vi "Node Status to gRPC Status.vi"(2 "Node Status":T10 {"Monitor Doubles"."4" format="%#_9g"; "Monitor Doubles"."3" format="%#_9g"; "Monitor Doubles"."2" format="%#_9g"; "Monitor Doubles"."1" format="%#_9g"}) -> (4 "gRPC Status":T1)   [LabVIEW 2021, in "CIFCoreCommon.lvlib"]
uses:
  CIFCoreCommon.lvlib
  Typedef/Plugin Status.ctl
  Typedef/Plugin State.ctl
  Typedef/Timing Statistics.ctl
  Typedef/Timing Stats Base.ctl
  Typedef/FIFO Statistics.ctl
  Typedef/Simple Error.ctl
  Typedef/Monitor Doubles.ctl
  Typedef/Monitor U64.ctl
  Typedef/Monitor I64.ctl
  Grpc/CIFCorePlugin_client/RPC Messages/cif_plugincore_StatusData.ctl
  Grpc/CIFCorePlugin_client/RPC Messages/cif_plugincore_StatusData_State.ctl
  Grpc/CIFCorePlugin_client/RPC Messages/cif_plugincore_TimingStatistics.ctl
  Grpc/CIFCorePlugin_client/RPC Messages/cif_plugincore_TimingStatsBasic.ctl
  Grpc/CIFCorePlugin_client/RPC Messages/cif_plugincore_FifoStatistics.ctl
  Grpc/CIFCorePlugin_client/RPC Messages/cif_plugincore_Error.ctl
  Grpc/CIFCorePlugin_client/RPC Messages/cif_plugincore_MonitorDoubles.ctl
  Grpc/CIFCorePlugin_client/RPC Messages/cif_plugincore_MonitorU64.ctl
  Grpc/CIFCorePlugin_client/RPC Messages/cif_plugincore_MonitorI64.ctl
  Grpc/CIFCorePlugin_client/CIFCorePlugin_client.lvlib
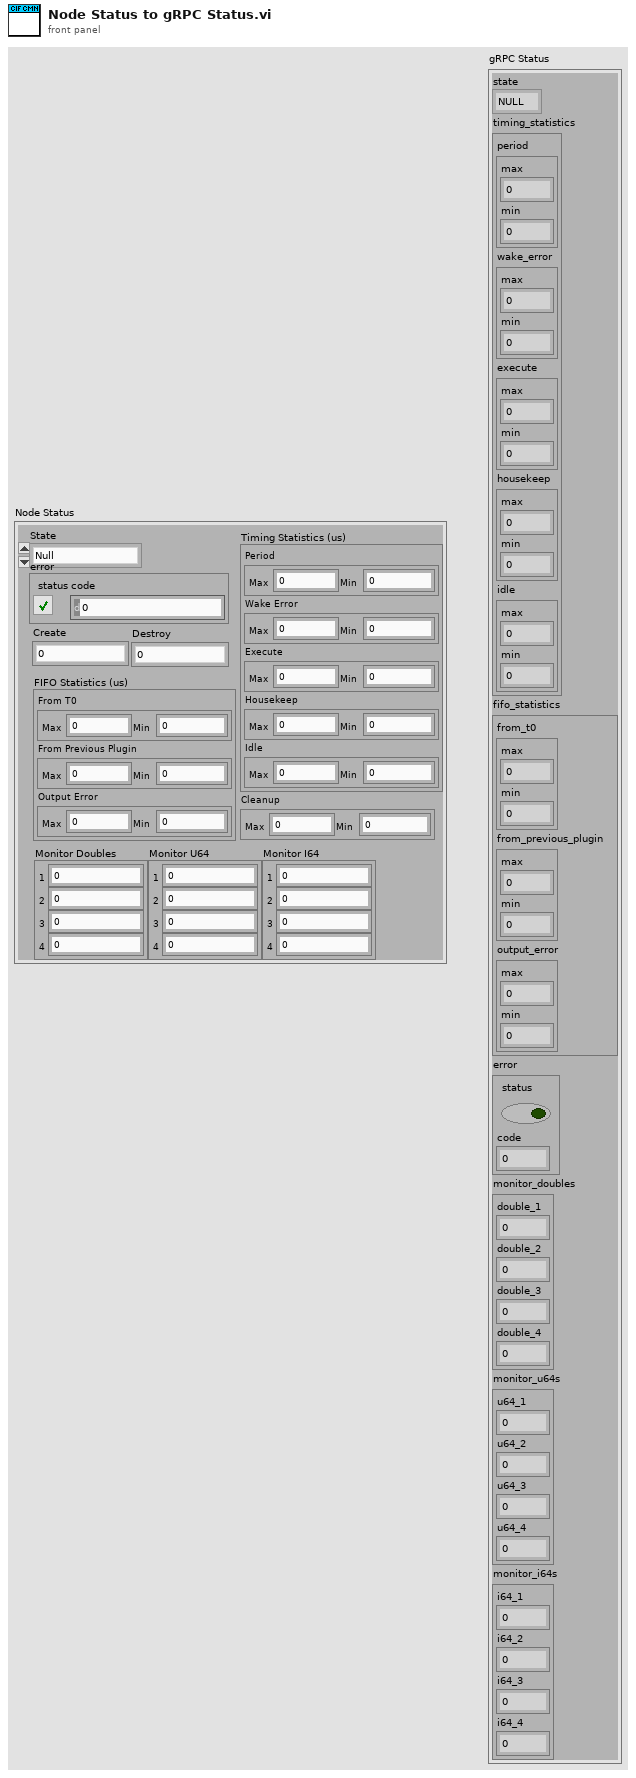
[diagram p1: front panel]
types:
  T1 = typedef "CIFCorePlugin_client.lvlib/cif_plugincore_StatusData.ctl" = cluster{"state":T2, "timing_statistics":T3, "fifo_statistics":T5, "error":T6, "monitor_doubles":T7, "monitor_u64s":T8, "monitor_i64s":T9}
  T2 = typedef "CIFCorePlugin_client.lvlib/cif_plugincore_StatusData_State.ctl" = enum32{"NULL", "CREATING", "LISTENING", "RUNNING", "CLEANINGUP", "DESTROYING"}
  T3 = typedef "CIFCorePlugin_client.lvlib/cif_plugincore_TimingStatistics.ctl" = cluster{"period":T4, "wake_error":T4, "execute":T4, "housekeep":T4, "idle":T4}
  T4 = typedef "CIFCorePlugin_client.lvlib/cif_plugincore_TimingStatsBasic.ctl" = cluster{"max":i32, "min":i32}
  T5 = typedef "CIFCorePlugin_client.lvlib/cif_plugincore_FifoStatistics.ctl" = cluster{"from_t0":T4, "from_previous_plugin":T4, "output_error":T4}
  T6 = typedef "CIFCorePlugin_client.lvlib/cif_plugincore_Error.ctl" = cluster{"status":bool, "code":i32}
  T7 = typedef "CIFCorePlugin_client.lvlib/cif_plugincore_MonitorDoubles.ctl" = cluster{"double_1":dbl, "double_2":dbl, "double_3":dbl, "double_4":dbl}
  T8 = typedef "CIFCorePlugin_client.lvlib/cif_plugincore_MonitorU64.ctl" = cluster{"u64_1":u64, "u64_2":u64, "u64_3":u64, "u64_4":u64}
  T9 = typedef "CIFCorePlugin_client.lvlib/cif_plugincore_MonitorI64.ctl" = cluster{"i64_1":i64, "i64_2":i64, "i64_3":i64, "i64_4":i64}
  T10 = typedef "CIFCoreCommon.lvlib/Plugin Status.ctl" = cluster{"State":T11, "Timing Statistics (us)":T12, "FIFO Statistics (us)":T14, "error":T15, "Monitor Doubles":T16, "Monitor U64":T17, "Monitor I64":T18, "Cleanup":T13, "Create":i32, "Destroy":i32}
  T11 = typedef "CIFCoreCommon.lvlib/Plugin State.ctl" = enum32{"Null", "Creating", "Listening", "Running", "CleaningUp", "Destroying"}
  T12 = typedef "CIFCoreCommon.lvlib/Timing Statistics.ctl" = cluster{"Period":T13, "Wake Error":T13, "Execute":T13, "Housekeep":T13, "Idle":T13}
  T13 = typedef "CIFCoreCommon.lvlib/Timing Stats Base.ctl" = cluster{"Max":i32, "Min":i32}
  T14 = typedef "CIFCoreCommon.lvlib/FIFO Statistics.ctl" = cluster{"From T0":T13, "From Previous Plugin":T13, "Output Error":T13}
  T15 = typedef "CIFCoreCommon.lvlib/Simple Error.ctl" = cluster{"status":bool, "code":i32}
  T16 = typedef "CIFCoreCommon.lvlib/Monitor Doubles.ctl" = cluster{"1":dbl, "2":dbl, "3":dbl, "4":dbl}
  T17 = typedef "CIFCoreCommon.lvlib/Monitor U64.ctl" = cluster{"1":u64, "2":u64, "3":u64, "4":u64}
  T18 = typedef "CIFCoreCommon.lvlib/Monitor I64.ctl" = cluster{"1":i64, "2":i64, "3":i64, "4":i64}
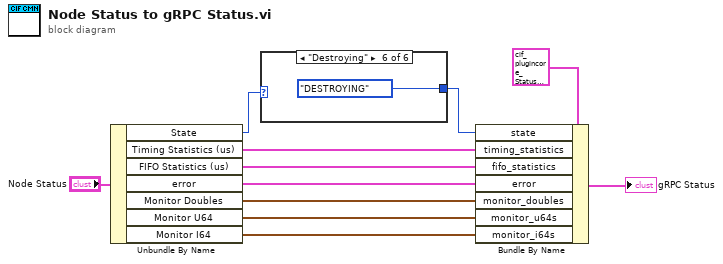
[diagram p0: block diagram]
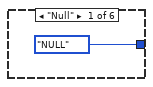
[diagram p2: hidden frame]
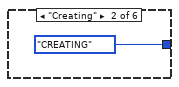
[diagram p3: hidden frame]
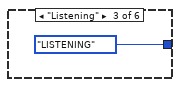
[diagram p4: hidden frame]
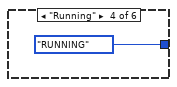
[diagram p5: hidden frame]
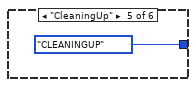
[diagram p6: hidden frame]
diagram:
  n1 = Unbundle By Name("Node Status") -> ("State"=w11:T11, "Timing Statistics (us)"=w10:T12, "FIFO Statistics (us)"=w9:T14, "error"=w8:T15, "Monitor Doubles"=w7:T16, "Monitor U64"=w6:T17, "Monitor I64"=w5:T18)
  n2 = case shown="\"Destroying\"" w11 {
    tunnel: [cif_plugincore_StatusData_State."NULL" ("state") cif_plugincore_StatusData_State."CREATING" ("state") cif_plugincore_StatusData_State."LISTENING" ("state") cif_plugincore_StatusData_State."RUNNING" ("state") cif_plugincore_StatusData_State."CLEANINGUP" ("state") cif_plugincore_StatusData_State."DESTROYING" ("state")] -> w1
    frame "Null" {
    }
    frame "Creating" {
    }
    frame "Listening" {
    }
    frame "Running" {
    }
    frame "CleaningUp" {
    }
    frame "Destroying" {
    }
  }
  n3 = Bundle By Name(cluster=T1 {"state"=enum."NULL", "timing_statistics"={"period"={"max"=0, "min"=0}, "wake_error"={"max"=0, "min"=0}, "execute"={"max"=0, "min"=0}, "housekeep"={"max"=0, "min"=0}, "idle"={"max"=0, "min"=0}}, "fifo_statistics"={"from_t0"={"max"=0, "min"=0}, "from_previous_plugin"={"max"=0, "min"=0}, "output_error"={"max"=0, "min"=0}}, "error"={"status"=FALSE, "code"=0}, "monitor_doubles"={"double_1"=0.0, "double_2"=0.0, "double_3"=0.0, "double_4"=0.0}, "monitor_u64s"={"u64_1"=0, "u64_2"=0, "u64_3"=0, "u64_4"=0}, "monitor_i64s"={"i64_1"=0, "i64_2"=0, "i64_3"=0, "i64_4"=0}} ("gRPC Status"), "state"=w1, "timing_statistics"=w10, "fifo_statistics"=w9, "error"=w8, "monitor_doubles"=w7, "monitor_u64s"=w6, "monitor_i64s"=w5) -> (→"gRPC Status":T1)
